vi "Renishaw-XL80_GetDX10Version.vi"(8 "error in (no error)":errorcluster, 11 "Renishaw-XL80_EMU in":refnum<class "Renishaw-XL80_EMU.lvclass">) -> (0 "error out":errorcluster, 2 "DX10Version":string, 3 "Renishaw-XL80_EMU out":refnum<class "Renishaw-XL80_EMU.lvclass">)   [LabVIEW 2024, in "Renishaw-XL80_EMU.lvclass"]
doc: "This read only property returns the version string of the DX10.\n\nDefinition\nHRESULTget_DX10Version( [out, retval] BSTR* pVal);\nParameters\npVal\nA variable that will be set to the version string of the DX10.\n\nComments\nThis property will return with an HRESULT of E_FAIL if the client has not previously connected to a DX10 by calling Connect.\n\nThe property will normally return an HRESULT of S_OK. However, it will return E_POINTER if the client supplies a null pointer for pVal, and in extremely low memory conditions it will return E_NOMEMORY."
uses:
  Renishaw-XL80_EMU.lvclass
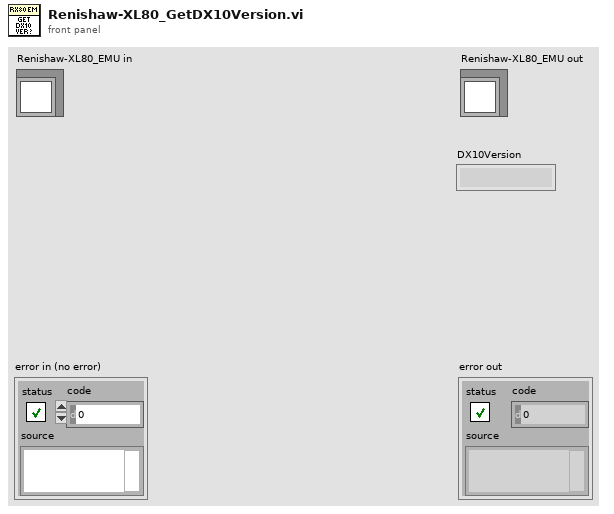
[diagram p1: front panel]
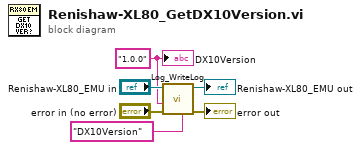
[diagram p0: block diagram]
diagram:
  w1 = "1.0.0" ("DX10Version")
  n1 = call-dynamic "Log_WriteLog.vi"("Additional text"="DX10Version", "error in (no error)"="error in (no error)", "Response"=w1, "Log in"="Renishaw-XL80_EMU in") -> ("error out"=→"error out":errorcluster, "Log out"=→"Renishaw-XL80_EMU out":refnum<class "Renishaw-XL80_EMU.lvclass">)  [unwired: 6 in]
  "DX10Version" <- w1
